vi "Example-IPS.vi"() -> ()   [LabVIEW 2013, in "Mercury iXX.lvlib"]
uses:
  <instrlib>/Mercury iXX/Mercury iXX.lvlib
  <instrlib>/Mercury iXX/Public/Libraries/Level Meter/Controls/Level Meter (Read).ctl
  <instrlib>/Mercury iXX/Public/Controls/Manufacturing Data.ctl
  <instrlib>/Mercury iXX/Public/Libraries/Level Meter/Controls/Nitrogen Configuration.ctl
  <instrlib>/Mercury iXX/Public/Libraries/Level Meter/Controls/Frequency Configuration.ctl
  <instrlib>/Mercury iXX/Public/Libraries/Level Meter/Controls/Signals.ctl
  <instrlib>/Mercury iXX/Public/Libraries/Level Meter/Controls/Helium Configuration.ctl
  <instrlib>/Mercury iXX/Public/Libraries/Level Meter/Controls/Resistance Configuration.ctl
  <instrlib>/Mercury iXX/Public/Libraries/Level Meter/Controls/Pre-Pulse.ctl
  <instrlib>/Mercury iXX/Public/Libraries/Level Meter/Controls/Pulse.ctl
  <instrlib>/Mercury iXX/Public/Libraries/Magnet/Controls/Device (Read).ctl
  <instrlib>/Mercury iXX/Public/Libraries/Magnet/Controls/Signals (Read).ctl
  <instrlib>/Mercury iXX/Public/Controls/Unit String.ctl
  <instrlib>/Mercury iXX/Public/Libraries/Magnet/Controls/Identifier.ctl
  <instrlib>/Mercury iXX/Public/Libraries/Temperature/Controls/Temperature Device (Read).ctl
  <instrlib>/Mercury iXX/Public/Libraries/Temperature/Controls/Temperature Sensor Type.ctl
  <instrlib>/Mercury iXX/Public/Libraries/Temperature/Controls/Excitation Cluster.ctl
  <instrlib>/Mercury iXX/Public/Libraries/Temperature/Controls/Excitation Type.ctl
  <instrlib>/Mercury iXX/Public/Libraries/Temperature/Controls/Calibration Cluster.ctl
  <instrlib>/Mercury iXX/Public/Libraries/Temperature/Controls/Calibration Interpolation.ctl
  <instrlib>/Mercury iXX/Public/Libraries/Temperature/Controls/Loop Cluster.ctl
  <instrlib>/Mercury iXX/Public/Libraries/Temperature/Controls/Temperature Signals Cluster.ctl
  <instrlib>/Mercury iXX/Public/Controls/Comms Transport Layer.ctl
  <instrlib>/Mercury iXX/Public/Libraries/System/Open/Open System.vi
  <instrlib>/Mercury iXX/Public/Libraries/System/Read/Catalogue (Read).vi
  <instrlib>/Mercury iXX/Public/Libraries/Temperature/Open/Open Temperature Device.vi
  <instrlib>/Mercury iXX/Public/Libraries/Temperature/Configuration/Read/Serial Number (Read).vi
  <instrlib>/Mercury iXX/Public/Libraries/Temperature/Configuration/Read/Nickname (Read).vi
  <instrlib>/Mercury iXX/Public/Libraries/Temperature/Configuration/Read/Excitation Magnitude (Read).vi
  <instrlib>/Mercury iXX/Public/Libraries/Temperature/Configuration/Read/Temperature Sensor (Read).vi
  <instrlib>/Mercury iXX/Public/Libraries/Temperature/Configuration/Read/Excitation Type (Read).vi
  <instrlib>/Mercury iXX/Public/Libraries/Temperature/Configuration/Read/Calibration Hot Limit (Read).vi
  <instrlib>/Mercury iXX/Public/Libraries/Temperature/Configuration/Read/Calibration Cold Limit (Read).vi
  <instrlib>/Mercury iXX/Public/Libraries/Pressure/Signals/Read/Current (Read).vi
  <instrlib>/Mercury iXX/Public/Libraries/Temperature/Signals/Read/Temperature (Read).vi
  <instrlib>/Mercury iXX/Public/Libraries/Temperature/Configuration/Read/Temperature Device (Read).vi
  <instrlib>/Mercury iXX/Public/Libraries/Control Loop/Configuration/Read/Control Loop (Read).vi
  <instrlib>/Mercury iXX/Public/Libraries/Level Meter/Open/Open Level Meter Device.vi
  <instrlib>/Mercury iXX/Public/Libraries/Level Meter/Configuration/Read/Level Meter Device (Read).vi
  <instrlib>/Mercury iXX/Public/Libraries/Level Meter/Configuration/Read/Serial Number (Read).vi
  <instrlib>/Mercury iXX/Public/Libraries/Level Meter/Configuration/Read/Helium Probe Resistance (Read).vi
  <instrlib>/Mercury iXX/Public/Libraries/Level Meter/Configuration/Read/Helium Pulse Mag (Read).vi
  <instrlib>/Mercury iXX/Public/Libraries/Level Meter/Configuration/Read/Helium Pulse Duration (Read).vi
  <instrlib>/Mercury iXX/Public/Libraries/Level Meter/Configuration/Read/Nitrogen Freq at 100 (Read).vi
  <instrlib>/Mercury iXX/Public/Libraries/Level Meter/Configuration/Read/Nitrogen Pulse Count Period (Read).vi
  <instrlib>/Mercury iXX/Public/Libraries/Level Meter/Signals/Read/Probe Resistance Helium (Read).vi
  <instrlib>/Mercury iXX/Public/Libraries/Level Meter/Signals/Read/Probe Level Helium (Read).vi
  <instrlib>/Mercury iXX/Public/Libraries/Level Meter/Signals/Read/Probe Count Nitrogen (Read).vi
  <instrlib>/Mercury iXX/Public/Libraries/Level Meter/Signals/Read/Probe Level Nitrogen (Read).vi
  <instrlib>/Mercury iXX/Public/Libraries/System/Read/Display Automatic Dimming (Read).vi
  <instrlib>/Mercury iXX/Public/Libraries/System/Read/Display Automatic Dimming Time (Read).vi
  <instrlib>/Mercury iXX/Public/Libraries/System/Read/Display Brightness (Read).vi
  <instrlib>/Mercury iXX/Public/Libraries/System/Read/Date (Read).vi
  <instrlib>/Mercury iXX/Public/Libraries/System/Read/Time (Read).vi
  <instrlib>/Mercury iXX/Public/Libraries/System/Read/DateTime (Read).vi
  <instrlib>/Mercury iXX/Public/Libraries/System/Read/HVer (Read).vi
  <instrlib>/Mercury iXX/Public/Libraries/System/Read/FVer (Read).vi
  <instrlib>/Mercury iXX/Public/Libraries/System/Read/Serial Number (Read).vi
  <instrlib>/Mercury iXX/Public/Libraries/System/Read/Flash Space (Read).vi
  <instrlib>/Mercury iXX/Public/Libraries/System/Read/Mode (Read).vi
  <instrlib>/Mercury iXX/Public/Libraries/Magnet/Open/Open Magnet Device.vi
  <instrlib>/Mercury iXX/Public/Libraries/Magnet/Configuration/Read/Magnet Device (Read).vi
  <instrlib>/Mercury iXX/Public/Libraries/Magnet/Configuration/Read/Serial Number (Read).vi
  <instrlib>/Mercury iXX/Public/Libraries/Magnet/Configuration/Read/Bipolar Output (Read).vi
  <instrlib>/Mercury iXX/Public/Libraries/Magnet/Configuration/Read/Output Configuration (Read).vi
  <instrlib>/Mercury iXX/Public/Libraries/Magnet/Configuration/Read/Current Limit (Read).vi
  <instrlib>/Mercury iXX/Public/Libraries/Magnet/Configuration/Read/Current to Field Factor (Read).vi
  <instrlib>/Mercury iXX/Public/Libraries/Magnet/Configuration/Read/Switch Present (Read).vi
  <instrlib>/Mercury iXX/Public/Libraries/Magnet/Configuration/Read/Software Voltage Limit (Read).vi
  <instrlib>/Mercury iXX/Public/Libraries/Magnet/Signals/Read/Current Rate (Read).vi
  <instrlib>/Mercury iXX/Public/Libraries/Magnet/Configuration/Read/PSU Action Status (Read).vi
  <instrlib>/Mercury iXX/Public/Libraries/System/Set/DateTime (Set).vi
  <instrlib>/Mercury iXX/Public/Libraries/System.lvlib
  <instrlib>/Mercury iXX/Public/Libraries/Level Meter.lvlib
  <instrlib>/Mercury iXX/Public/Libraries/Magnet.lvlib
  <instrlib>/Mercury iXX/Public/Libraries/Temperature.lvlib
  <instrlib>/Mercury iXX/Public/Libraries/Pressure.lvlib
  <instrlib>/Mercury iXX/Public/Libraries/Control Loop.lvlib
panel:
  in  "Mercury Functions":T1(tab)
  out "time stamp":timestamp=timestamp(3542718986 s since 1904-01-01)
  out "Free Space":i32=166152 caption="Free Space (KB)"
  out "Set Date Response":string="VALID"
  out "String":string="NORM" caption="User Mode"
  out "Date":string="2016:04:05"
  out "Time":string="11:36:26"
  out "Hardware Version":string="65"
  out "Firmware Version":string="2.2.6.20"
  out "Serial Number":string="153350063"
  out "Devices":string[](array[string])=["DB3.L1:LVL", "GRPX:PSU", "GRPY:PSU", "GRPZ:PSU", "MB1.T1:TEMP", "PSU.M1:PSU", "PSU.M2:PSU", "PSU.M3:PSU"]
  out "S/W Version(s)":string[](array[string])=["2.2.6.20\n"]
  out "Serial Number(s)":string[](array[string])=["153350063"]
  out "# of Instruments":i32=1
  out "Automatic Dimming":string="OFF"
  out "Dimming Time":string="5"
  out "Display Brightness":string="100"
  in  "ITC IP Address":string="130.49.180.102"
  out "LVL Device DetailSettings":T2
  out "LVL S/N":string
  out "LVL P Magnitude":dbl=-inf caption="Pulse Magnitude (mA)"
  out "LVL P Duration":dbl=-inf caption="Pulse Duration (s)"
  out "N Freq 100%":dbl=-inf caption="Frequency at 100% (Hz)"
  out "N Pulse Period":dbl=-inf caption="Pulse Period (ms)"
  out "He Res Config":T8
  out "He Resistance":dbl=-inf caption="Resistance (Ohms)"
  out "He Level":dbl=-inf caption="Helium Level (%)"
  out "N Counter":u32 caption="Counter"
  out "N Level":dbl=-inf caption="Nitrogen Level (%)"
  out "Excitation Magnitude":dbl=5.0
  out "Sensor Type":string="NTC"
  out "Excitation Type":string="UNIP"
  out "Hot Limit":dbl=1000.0
  out "H Unit":T11="K"
  out "Cold Limit":dbl=1000.0
  out "C Unit":T11="K"
  out "Unit":T11
  out "Voltage":dbl=0.005
  out "V Unit":T11="V"
  out "Temperature":dbl=1.93
  out "T Unit":T11="K"
  out "Temperature Device Settings":T12={"Manufacturing"={"Hardware Version"="65", "Firmware Version"="2.2", "Serial Number"="154650110"}, "Temperature Sensor Type"="NTC", "Excitation"={"Excitation Type"="UNIP", "Magnitude"="5.00"}, "Calibration"={"Filename"="59543_iTC-lambda.dat", "Interpolation"="LIN", "Scaling Factor"="1", "Offset Factor"="0", "Hot Limit"="1000.00K", "Cold Limit"="1000.00K", "Last Calibration"="", "Reference"="Internal"}, "Control Loop"={"Heater"="", "Auxiliary"="", "Heater Auto"="", "Percentage Heat"="", "Temperature Set Point"="", "PID Auto (from file)"="", "P Value"="", "I Value"="", "D Value"="", "Auto PID Table Filename"="", "Flow Auto"="", "Target Heater Table"="", "Sweep mode"="", "Sweep Table Filename"="", "Percentage Flow"=""}, "Temperature Signals"={"Voltage"="5.0000mV", "Current"="0.0005µA", "Power"="0.0000µW", "Resistance"="10000000.0000R", "Temperature"="1.9300K", "Sensitivity"="5181347.1503R/K", "Reference"="N/A"}, "Nickname"="Mag_AB_MB1", "Status"="2"}
  out "Temp S/N":string="154650110"
  out "T Nickname":string="Mag_AB_MB1"
  out "T Loop Details":T18
  out "Magnet Device Details":T20={"Manufacturing"={"Hardware Version"="65", "Firmware Version"="2.4", "Serial Number"="151250009"}, "Nickname"="PSU.M1", "Bipolar Output"="ON", "String"="NOT_FOUND", "Current Limit"=58.0, "AtoB"=1.0, "Inductance"=39.406, "Switch Present"="NOT_FOUND", "Swh Htr Current"=86.0, "SW VLIM"=9.0, "V Trans Time"=1000.0, "Magnet PSU Signals"={"Voltage"=-0.0003, "Current"=0.0002, "Current Rate"=0.0, "Field"=0.0, "Field Rate"=0.0, "Persistant Current"=0.0, "Persistant Field"=0.0, "Target Current"=0.0, "Target Field"=0.0, "Target Current Rate"=0.0, "Target Field Rate"=0.0, "Switch Heater Status (SWHT)"="NOT_FOUND", "Switch Heater Status (SWHN)"="NOT_FOUND"}, "PSU Action"="NOT_FOUND", "Status"="4000", "Level Limit"=0.0, "Temperature Limit"=0.0} {"Temperature Limit" format="%#.1f"; "Level Limit" format="%#.1f"; "V Trans Time" format="%#.1f"; "SW VLIM" format="%#.1f"; "Swh Htr Current" format="%#.1f"; "Inductance" format="%#.1f"; "AtoB" format="%#.1f"; "Current Limit" format="%#.1f"}
  out "Mag S/N":string="151250009"
  out "Bipolar Output":string="ON"
  out "Out Config":string="NOT_FOUND" caption="Output Configuration"
  out "Current Limit":dbl=58.0 caption="Current Limit (A)" format="%#.1f"
  out "AtoB":dbl=1.0 caption="Current Field Factor (A/T)" format="%#.1f"
  out "Switch Present":string="NOT_FOUND"
  out "SW VLIM":dbl=9.0 caption="Software Voltage Limit (V)" format="%#.1f"
  out "Unit 8":T11
  out "Unit 9":T11
  out "Unit 10":T11
  out "Current Rate":dbl
  out "PSU Act Stat":string="NOT_FOUND" caption="PSU Action Status"
  out "Unit 11":T11
  in  "Device Identifier":T22="PSU.M1"
  # "IPS"
  # "101, 102, 67"
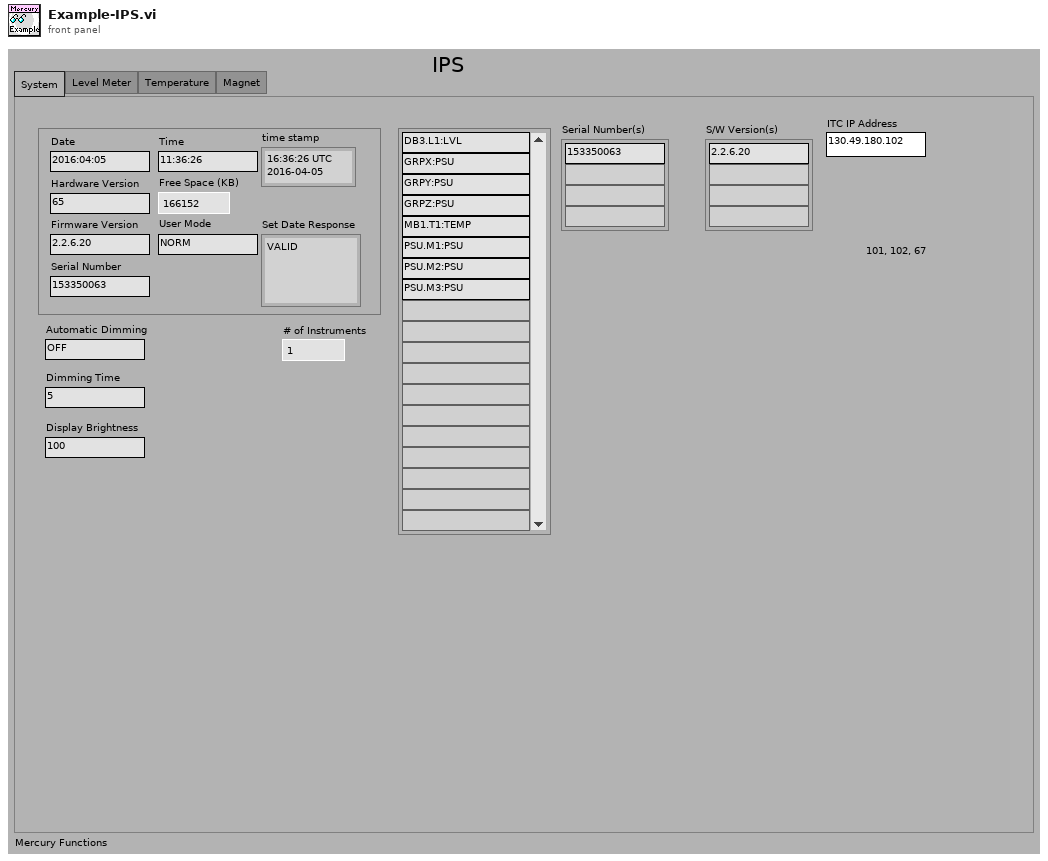
[diagram p1: front panel]
types:
  T1 = enum32{"System", "Level Meter", "Temperature", "Magnet"}
  T2 = typedef "Mercury iXX.lvlib/Level Meter.lvlib/Level Meter (Read).ctl" = cluster{"Manufacturing":T3, "Nitrogen Configuration":T4, "Signals":T6, "Nickname":string, "Status":string, "Helium Configuration":T7}
  T3 = typedef "Mercury iXX.lvlib/Manufacturing Data.ctl" = cluster{"Hardware Version":string, "Firmware Version":string, "Serial Number":string}
  T4 = typedef "Mercury iXX.lvlib/Level Meter.lvlib/Nitrogen Configuration.ctl" = cluster{"Frequency Configuration":T5, "Pulse Period":dbl}
  T5 = typedef "Mercury iXX.lvlib/Level Meter.lvlib/Frequency Configuration.ctl" = cluster{"Freq 0%":dbl, "Freq 100%":dbl}
  T6 = typedef "Mercury iXX.lvlib/Level Meter.lvlib/Signals.ctl" = cluster{"Helium Signals":cluster{"Resistance":dbl, "Level":dbl}, "Nitrogen Signals":cluster{"Count":dbl, "Freq":dbl, "Level":dbl}}
  T7 = typedef "Mercury iXX.lvlib/Level Meter.lvlib/Helium Configuration.ctl" = cluster{"Resistance Configuration":T8, "Pre-Pulse":T9, "Pulse":T10}
  T8 = typedef "Mercury iXX.lvlib/Level Meter.lvlib/Resistance Configuration.ctl" = cluster{"Res 0%":dbl, "Res 100%":dbl}
  T9 = typedef "Mercury iXX.lvlib/Level Meter.lvlib/Pre-Pulse.ctl" = cluster{"Magnitude":dbl, "Duration":dbl}
  T10 = typedef "Mercury iXX.lvlib/Level Meter.lvlib/Pulse.ctl" = cluster{"Magnitude":dbl, "Duration":dbl, "Delay":dbl}
  T11 = typedef "Mercury iXX.lvlib/Unit String.ctl" = string
  T12 = typedef "Mercury iXX.lvlib/Temperature.lvlib/Temperature Device (Read).ctl" = cluster{"Manufacturing":T3, "Temperature Sensor Type":T13, "Excitation":T14, "Calibration":T16, "Control Loop":T18, "Temperature Signals":T19, "Nickname":string, "Status":string}
  T13 = typedef "Mercury iXX.lvlib/Temperature.lvlib/Temperature Sensor Type.ctl" = string
  T14 = typedef "Mercury iXX.lvlib/Temperature.lvlib/Excitation Cluster.ctl" = cluster{"Excitation Type":T15, "Magnitude":string}
  T15 = typedef "Mercury iXX.lvlib/Temperature.lvlib/Excitation Type.ctl" = string
  T16 = typedef "Mercury iXX.lvlib/Temperature.lvlib/Calibration Cluster.ctl" = cluster{"Filename":string, "Interpolation":T17, "Scaling Factor":string, "Offset Factor":string, "Hot Limit":string, "Cold Limit":string, "Last Calibration":string, "Reference":string}
  T17 = typedef "Mercury iXX.lvlib/Temperature.lvlib/Calibration Interpolation.ctl" = string
  T18 = typedef "Mercury iXX.lvlib/Temperature.lvlib/Loop Cluster.ctl" = cluster{"Heater":string, "Auxiliary":string, "Heater Auto":string, "Percentage Heat":string, "Temperature Set Point":string, "PID Auto (from file)":string, "P Value":string, "I Value":string, "D Value":string, "Auto PID Table Filename":string, "Flow Auto":string, "Target Heater Table":string, "Sweep mode":string, "Sweep Table Filename":string, "Percentage Flow":string}
  T19 = typedef "Mercury iXX.lvlib/Temperature.lvlib/Temperature Signals Cluster.ctl" = cluster{"Voltage":string, "Current":string, "Power":string, "Resistance":string, "Temperature":string, "Sensitivity":string, "Reference":string}
  T20 = typedef "Mercury iXX.lvlib/Magnet.lvlib/Device (Read).ctl" = cluster{"Manufacturing":T3, "Nickname":string, "Bipolar Output":string, "String":string, "Current Limit":dbl, "AtoB":dbl, "Inductance":dbl, "Switch Present":string, "Swh Htr Current":dbl, "SW VLIM":dbl, "V Trans Time":dbl, "Magnet PSU Signals":T21, "PSU Action":string, "Status":string, "Level Limit":dbl, "Temperature Limit":dbl}
  T21 = typedef "Mercury iXX.lvlib/Magnet.lvlib/Signals (Read).ctl" = cluster{"Voltage":dbl, "Current":dbl, "Current Rate":dbl, "Field":dbl, "Field Rate":dbl, "Persistant Current":dbl, "Persistant Field":dbl, "Target Current":dbl, "Target Field":dbl, "Target Current Rate":dbl, "Target Field Rate":dbl, "Switch Heater Status (SWHT)":string, "Switch Heater Status (SWHN)":string}
  T22 = typedef "Mercury iXX.lvlib/Magnet.lvlib/Identifier.ctl" = string
  T23 = typedef "Mercury iXX.lvlib/Comms Transport Layer.ctl" = enum16{"Ethernet TCP/IP", "USB", "ISOBus - RS-232", "GPIB"}
  T24 = typedef "Mercury iXX.lvlib/Mercury Reference.ctl" = cluster{"Comms":refnum<visa-resource-name>, "Device ID":string[], "Comms Layer":T23, "Command":string, "Query reference":T25}
  T25 = typedef "Mercury iXX.lvlib/Query Dynamic Reference.ctl" = refnum<vi>
  T26 = typedef "Mercury iXX.lvlib/Magnet.lvlib/Output Configuration.ctl" = string
  T27 = typedef "Mercury iXX.lvlib/Magnet.lvlib/PSU Actions.ctl" = string
  T28 = typedef "Mercury iXX.lvlib/System.lvlib/User Mode.ctl" = string
  T29 = typedef "Mercury iXX.lvlib/Response String.ctl" = string
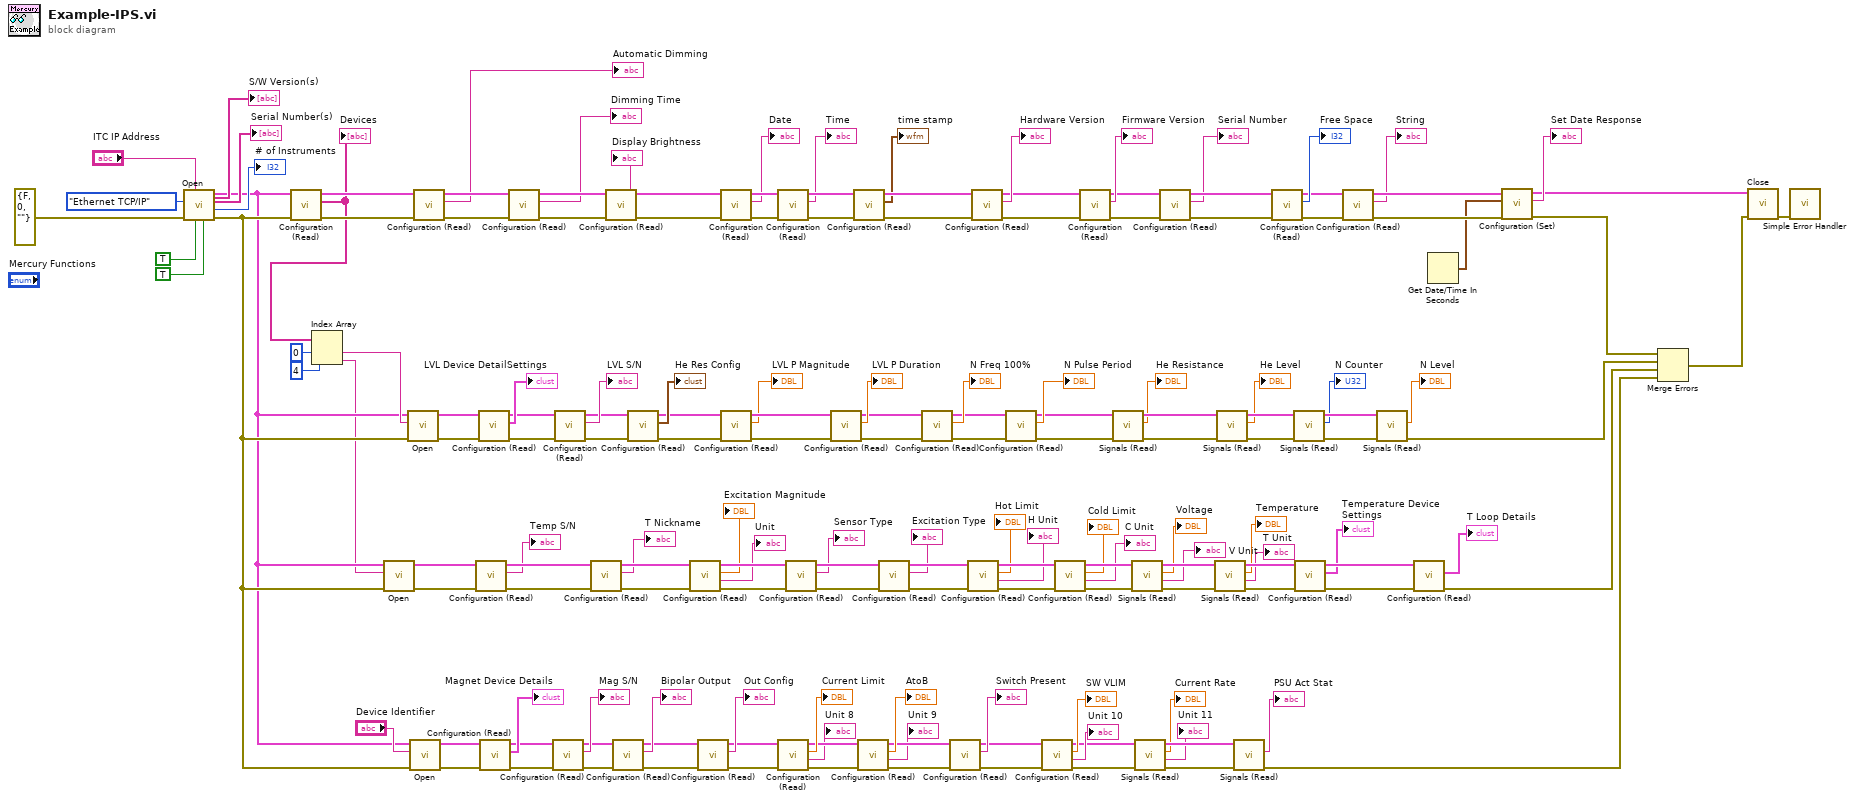
[diagram p0: block diagram]
diagram:
  n1 = call-poly <instrlib>:"Open.vi"("Clear Previous Connections (False)"=TRUE ("Clear Previous Connections (True)"), "ID Query (True)"=TRUE, "IP Address"="ITC IP Address", "error in (no error)"=errorcluster {"status"=FALSE, "code"=0, "source"=""}, "Comms Layer"=Comms_Transport_Layer."Ethernet TCP/IP") -> ("error out"=w32:errorcluster, "# of Instruments"=→"# of Instruments":i32, "Serial Number(s)"=→"Serial Number(s)":string[], "Mercury Reference Out"=w31:T24, "S/W Version(s)"=→"S/W Version(s)":string[])  [unwired: 2 in]
  n2 = call-poly <instrlib>:"Configuration (Read).vi"("error in"=w32, "Mercury Reference In"=w31) -> ("error out"=w85:errorcluster, "Devices"=w30:string[], "Mercury Reference Out"=w84:T24)  [unwired: 1 in, 6 out]
  "Devices" <- w30
  n3 = Index Array(array=w30, index #1=0 ("index"), index #2=4 ("index")) -> (element #1=w147:string, element #2=w1:string)
  n4 = call-poly <instrlib>:"Open.vi"("error in (no error)"=w32, "Device Identifier"=w1, "Mercury Reference In"=w31) -> ("error out"=w33:errorcluster, "Mercury Reference Out"=w29:T24)  [unwired: 7 out]
  n5 = call-poly <instrlib>:"Open.vi"("error in (no error)"=w32, "Device Identifier"=w147, "Mercury Reference In"=w31) -> ("error out"=w136:errorcluster, "Mercury Reference Out"=w137:T24)  [unwired: 7 out]
  n6 = call-poly <instrlib>:"Open.vi"("error in (no error)"=w32, "Device Identifier"="Device Identifier", "Mercury Reference In"=w31) -> ("error out"=w80:errorcluster, "Mercury Reference Out"=w81:T24)  [unwired: 7 out]
  n7 = call-poly <instrlib>:"Configuration (Read).vi"("error in"=w85, "Mercury Reference In"=w84) -> ("error out"=w92:errorcluster, "Automatic Dimming"=→"Automatic Dimming":string, "Mercury Reference Out"=w91:T24)  [unwired: 1 in, 6 out]
  n8 = call-poly <instrlib>:"Configuration (Read).vi"("error in"=w33, "Mercury Reference In"=w29) -> ("error out"=w43:errorcluster, "Serial Number"=→"Temp S/N":string, "Mercury Reference Out"=w28:T24)  [unwired: 1 in, 6 out]
  n9 = call-poly <instrlib>:"Configuration (Read).vi"("error in"=w136, "Mercury Reference In"=w137) -> ("error out"=w131:errorcluster, "LVL Device Settings"=→"LVL Device DetailSettings":T2, "Mercury Reference Out"=w134:T24)  [unwired: 1 in, 6 out]
  n10 = call-poly <instrlib>:"Configuration (Read).vi"("error in"=w80, "Mercury Reference In"=w81) -> ("error out"=w77:errorcluster, "Magnet Device Details"=→"Magnet Device Details":T20, "Mercury Reference Out"=w78:T24)  [unwired: 1 in, 6 out]
  n11 = call-poly <instrlib>:"Configuration (Read).vi"("error in"=w92, "Mercury Reference In"=w91) -> ("error out"=w89:errorcluster, "Dimming Time"=→"Dimming Time":string, "Mercury Reference Out"=w90:T24)  [unwired: 1 in, 6 out]
  n12 = call-poly <instrlib>:"Configuration (Read).vi"("error in"=w77, "Mercury Reference In"=w78) -> ("error out"=w74:errorcluster, "Serial Number"=→"Mag S/N":string, "Mercury Reference Out"=w75:T24)  [unwired: 1 in, 6 out]
  n13 = call-poly <instrlib>:"Configuration (Read).vi"("error in"=w131, "Mercury Reference In"=w134) -> ("error out"=w130:errorcluster, "Serial Number"=→"LVL S/N":string, "Mercury Reference Out"=w132:T24)  [unwired: 1 in, 6 out]
  n14 = call-poly <instrlib>:"Configuration (Read).vi"("error in"=w43, "Mercury Reference In"=w28) -> ("error out"=w42:errorcluster, "Nickname"=→"T Nickname":string, "Mercury Reference Out"=w27:T24)  [unwired: 1 in, 6 out]
  n15 = call-poly <instrlib>:"Configuration (Read).vi"("error in"=w89, "Mercury Reference In"=w90) -> ("error out"=w83:errorcluster, "Display Brightness"=→"Display Brightness":string, "Mercury Reference Out"=w82:T24)  [unwired: 1 in, 6 out]
  n16 = call-poly <instrlib>:"Configuration (Read).vi"("error in"=w74, "Mercury Reference In"=w75) -> ("error out"=w71:errorcluster, "Bipolar Output"=→"Bipolar Output":string, "Mercury Reference Out"=w72:T24)  [unwired: 1 in, 6 out]
  n17 = call-poly <instrlib>:"Configuration (Read).vi"("error in"=w130, "Mercury Reference In"=w132) -> ("error out"=w127:errorcluster, "Resistance Configuration"=→"He Res Config":T8, "Mercury Reference Out"=w128:T24)  [unwired: 1 in, 6 out]
  n18 = call-poly <instrlib>:"Configuration (Read).vi"("error in"=w42, "Mercury Reference In"=w27) -> ("error out"=w41:errorcluster, "Unit"=→"Unit":T11, "Excitation Magnitude"=→"Excitation Magnitude":dbl, "Mercury Reference Out"=w26:T24)  [unwired: 1 in, 5 out]
  n19 = call-poly <instrlib>:"Configuration (Read).vi"("error in"=w71, "Mercury Reference In"=w72) -> ("error out"=w68:errorcluster, "Out Config"=→"Out Config":T26, "Mercury Reference Out"=w69:T24)  [unwired: 1 in, 6 out]
  n20 = call-poly <instrlib>:"Configuration (Read).vi"("error in"=w83, "Mercury Reference In"=w82) -> ("error out"=w164:errorcluster, "Date"=→"Date":string, "Mercury Reference Out"=w165:T24)  [unwired: 1 in, 6 out]
  n21 = call-poly <instrlib>:"Configuration (Read).vi"("error in"=w127, "Mercury Reference In"=w128) -> ("error out"=w125:errorcluster, "Magnitude"=→"LVL P Magnitude":dbl, "Mercury Reference Out"=w126:T24)  [unwired: 1 in, 6 out]
  n22 = call-poly <instrlib>:"Configuration (Read).vi"("error in"=w164, "Mercury Reference In"=w165) -> ("error out"=w162:errorcluster, "Time"=→"Time":string, "Mercury Reference Out"=w163:T24)  [unwired: 1 in, 6 out]
  n23 = call-poly <instrlib>:"Configuration (Read).vi"("error in"=w68, "Mercury Reference In"=w69) -> ("error out"=w65:errorcluster, "Unit"=→"Unit 8":T11, "Current Limit"=→"Current Limit":dbl, "Mercury Reference Out"=w66:T24)  [unwired: 1 in, 5 out]
  n24 = call-poly <instrlib>:"Configuration (Read).vi"("error in"=w41, "Mercury Reference In"=w26) -> ("error out"=w40:errorcluster, "Sensor Type"=→"Sensor Type":T13, "Mercury Reference Out"=w25:T24)  [unwired: 1 in, 6 out]
  n25 = call-poly <instrlib>:"Configuration (Read).vi"("error in"=w125, "Mercury Reference In"=w126) -> ("error out"=w121:errorcluster, "Duration"=→"LVL P Duration":dbl, "Mercury Reference Out"=w122:T24)  [unwired: 1 in, 6 out]
  n26 = call-poly <instrlib>:"Configuration (Read).vi"("error in"=w162, "Mercury Reference In"=w163) -> ("error out"=w160:errorcluster, "time stamp"=→"time stamp":timestamp, "Mercury Reference Out"=w161:T24)  [unwired: 1 in, 6 out]
  n27 = call-poly <instrlib>:"Configuration (Read).vi"("error in"=w65, "Mercury Reference In"=w66) -> ("error out"=w62:errorcluster, "Unit"=→"Unit 9":T11, "AtoB"=→"AtoB":dbl, "Mercury Reference Out"=w63:T24)  [unwired: 1 in, 5 out]
  n28 = call-poly <instrlib>:"Configuration (Read).vi"("error in"=w40, "Mercury Reference In"=w25) -> ("error out"=w39:errorcluster, "Excitation Type"=→"Excitation Type":T15, "Mercury Reference Out"=w24:T24)  [unwired: 1 in, 6 out]
  n29 = call-poly <instrlib>:"Configuration (Read).vi"("error in"=w121, "Mercury Reference In"=w122) -> ("error out"=w118:errorcluster, "Freq 100%"=→"N Freq 100%":dbl, "Mercury Reference Out"=w119:T24)  [unwired: 1 in, 6 out]
  n30 = call-poly <instrlib>:"Configuration (Read).vi"("error in"=w62, "Mercury Reference In"=w63) -> ("error out"=w59:errorcluster, "Switch Present"=→"Switch Present":string, "Mercury Reference Out"=w60:T24)  [unwired: 1 in, 6 out]
  n31 = call-poly <instrlib>:"Configuration (Read).vi"("error in"=w39, "Mercury Reference In"=w24) -> ("error out"=w38:errorcluster, "Unit"=→"H Unit":T11, "Hot Limit"=→"Hot Limit":dbl, "Mercury Reference Out"=w23:T24)  [unwired: 1 in, 5 out]
  n32 = call-poly <instrlib>:"Configuration (Read).vi"("error in"=w160, "Mercury Reference In"=w161) -> ("error out"=w94:errorcluster, "Hardware Version"=→"Hardware Version":string, "Mercury Reference Out"=w95:T24)  [unwired: 1 in, 6 out]
  n33 = call-poly <instrlib>:"Configuration (Read).vi"("error in"=w118, "Mercury Reference In"=w119) -> ("error out"=w115:errorcluster, "Pulse Period"=→"N Pulse Period":dbl, "Mercury Reference Out"=w116:T24)  [unwired: 1 in, 6 out]
  n34 = call-poly <instrlib>:"Configuration (Read).vi"("error in"=w59, "Mercury Reference In"=w60) -> ("error out"=w53:errorcluster, "Unit"=→"Unit 10":T11, "SW VLIM"=→"SW VLIM":dbl, "Mercury Reference Out"=w54:T24)  [unwired: 1 in, 5 out]
  n35 = call-poly <instrlib>:"Configuration (Read).vi"("error in"=w38, "Mercury Reference In"=w23) -> ("error out"=w37:errorcluster, "Unit"=→"C Unit":T11, "Cold Limit"=→"Cold Limit":dbl, "Mercury Reference Out"=w22:T24)  [unwired: 1 in, 5 out]
  n36 = call-poly <instrlib>:"Configuration (Read).vi"("error in"=w94, "Mercury Reference In"=w95) -> ("error out"=w96:errorcluster, "Firmware Version"=→"Firmware Version":string, "Mercury Reference Out"=w97:T24)  [unwired: 1 in, 6 out]
  n37 = call-poly <instrlib>:"Signals (Read).vi"("error in"=w115, "Mercury Reference In"=w116) -> ("error out"=w113:errorcluster, "Resistance"=→"He Resistance":dbl, "Mercury Reference Out"=w114:T24)  [unwired: 1 in, 6 out]
  n38 = call-poly <instrlib>:"Signals (Read).vi"("error in"=w37, "Mercury Reference In"=w22) -> ("error out"=w36:errorcluster, "Unit"=→"V Unit":T11, "Current"=→"Voltage":dbl, "Mercury Reference Out"=w21:T24)  [unwired: 1 in, 5 out]
  n39 = call-poly <instrlib>:"Signals (Read).vi"("error in"=w53, "Mercury Reference In"=w54) -> ("error out"=w51:errorcluster, "Unit"=→"Unit 11":T11, "Current Rate"=→"Current Rate":dbl, "Mercury Reference Out"=w52:T24)  [unwired: 1 in, 5 out]
  n40 = call-poly <instrlib>:"Configuration (Read).vi"("error in"=w96, "Mercury Reference In"=w97) -> ("error out"=w158:errorcluster, "Serial Number"=→"Serial Number":string, "Mercury Reference Out"=w159:T24)  [unwired: 1 in, 6 out]
  n41 = call-poly <instrlib>:"Signals (Read).vi"("error in"=w36, "Mercury Reference In"=w21) -> ("error out"=w35:errorcluster, "Unit"=→"T Unit":T11, "Temperature"=→"Temperature":dbl, "Mercury Reference Out"=w20:T24)  [unwired: 1 in, 5 out]
  n42 = call-poly <instrlib>:"Signals (Read).vi"("error in"=w113, "Mercury Reference In"=w114) -> ("error out"=w111:errorcluster, "Level"=→"He Level":dbl, "Mercury Reference Out"=w112:T24)  [unwired: 1 in, 6 out]
  n43 = call-poly <instrlib>:"Signals (Read).vi"("error in"=w51, "Mercury Reference In"=w52) -> ("error out"=w44:errorcluster, "PSU Act Stat"=→"PSU Act Stat":T27)  [unwired: 1 in, 7 out]
  n44 = call-poly <instrlib>:"Configuration (Read).vi"("error in"=w158, "Mercury Reference In"=w159) -> ("error out"=w145:errorcluster, "Free Space"=→"Free Space":i32, "Mercury Reference Out"=w146:T24)  [unwired: 1 in, 6 out]
  n45 = call-poly <instrlib>:"Signals (Read).vi"("error in"=w111, "Mercury Reference In"=w112) -> ("error out"=w109:errorcluster, "Counter"=→"N Counter":u32, "Mercury Reference Out"=w110:T24)  [unwired: 1 in, 6 out]
  n46 = call-poly <instrlib>:"Configuration (Read).vi"("error in"=w35, "Mercury Reference In"=w20) -> ("error out"=w34:errorcluster, "Device Details"=→"Temperature Device Settings":T12, "Mercury Reference Out"=w19:T24)  [unwired: 1 in, 6 out]
  n47 = call-poly <instrlib>:"Configuration (Read).vi"("error in"=w145, "Mercury Reference In"=w146) -> ("error out"=w153:errorcluster, "Mode"=→"String":T28, "Mercury Reference Out"=w152:T24)  [unwired: 1 in, 6 out]
  n48 = call-poly <instrlib>:"Signals (Read).vi"("error in"=w109, "Mercury Reference In"=w110) -> ("error out"=w45:errorcluster, "Level"=→"N Level":dbl)  [unwired: 1 in, 7 out]
  n49 = call-poly <instrlib>:"Configuration (Read).vi"("error in"=w34, "Mercury Reference In"=w19) -> ("error out"=w18:errorcluster, "Loop Details"=→"T Loop Details":T18)  [unwired: 1 in, 7 out]
  n50 = Get Date/Time In Seconds() -> (seconds since 1Jan1904=w98:timestamp)
  n51 = call-poly <instrlib>:"Configuration (Set).vi"("error in"=w153, "time stamp"=w98, "Mercury Reference In"=w152) -> ("error out"=w46:errorcluster, "Response"=→"Set Date Response":T29, "Mercury Reference Out"=w93:T24)  [unwired: 1 in, 5 out]
  n52 = Merge Errors(w46, w45, w18, w44) -> (w150:errorcluster)
  n53 = call <instrlib>:"Close.vi"("error in (no error)"=w150, "Mercury Reference"=w93) -> ("error out"=w101:errorcluster)  [unwired: 9 out]
  n54 = call <vilib>:"Simple Error Handler.vi"("error in (no error)"=w101) -> ()  [unwired: 1 in, 8 out]
